vi "Set Template Dut Results.vi"(8 "error in (no error)":errorcluster, 10 "Template Dut Results":T1, 11 "Template Dut in":refnum<class "Template Dut.lvclass">) -> (0 "error out":errorcluster, 3 "Template Dut out":refnum<class "Template Dut.lvclass">)   [LabVIEW 2015, in "niDTS Template.lvlib" / "Template Dut.lvclass"]
uses:
  Template Dut.lvclass
  Includes/Template Dut INC Results.ctl
  Template Dut.lvclass/Template Dut.ctl
  niDTS Template.lvlib
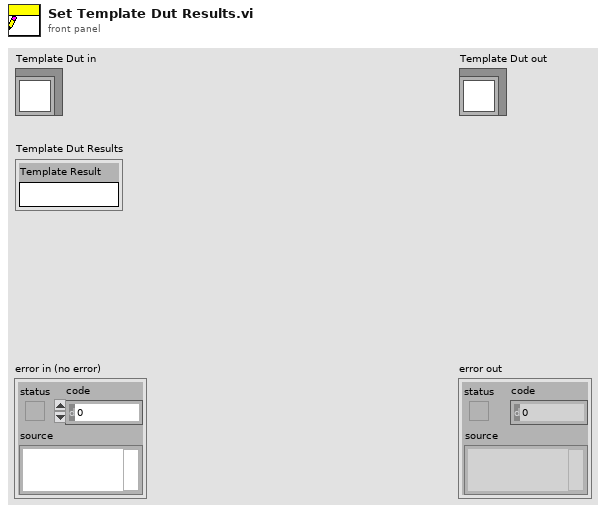
[diagram p1: front panel]
types:
  T1 = typedef "niDTS Template.lvlib/Template Dut INC Results.ctl" = cluster{"Template Result":string}
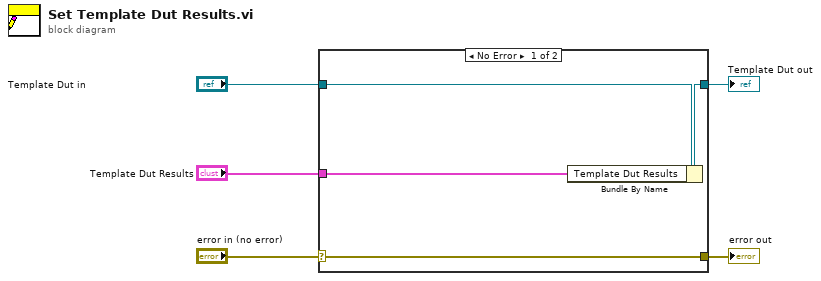
[diagram p0: block diagram]
diagram:
  n1 = case shown="No Error" "error in (no error)" {
    selector: "error in (no error)" -> [w9 w10]
    tunnel: [w9 w10] -> w4
    tunnel: [w7 w11] -> w2
    tunnel: "Template Dut in" -> [w8 w11]
    tunnel: "Template Dut Results" -> [w6 _]
    frame No Error {
      n2 = Bundle By Name(cluster=w8, "Template Dut Results"=w6) -> (w7:refnum<class "Template Dut.lvclass">)
    }
    frame Error {
    }
  }
  "error out" <- w4
  "Template Dut out" <- w2
